vi "Event Handle Loop_Mouse Up.vi"(8 "error in (no error)":errorcluster, 10 "Coords":T1, 11 "QMenu Class in":refnum<class "QMenu Class.lvclass">) -> (0 "error out":errorcluster, 3 "QMenu Class out":refnum<class "QMenu Class.lvclass">)   [LabVIEW 2020, in "QTab.lvlib" / "QMenu Class.lvclass"]
uses:
  QMenu Class.lvclass
  <vilib>/Utility/miscctls.llb/LVPoint32TypeDef.ctl
  QMenu Class.lvclass/QMenu Class.ctl
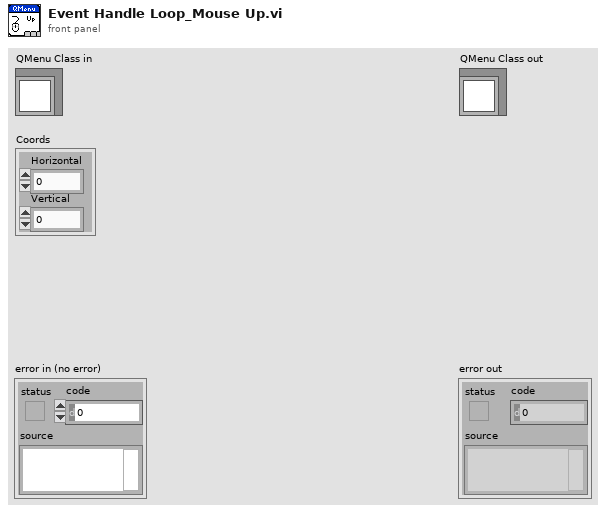
[diagram p1: front panel]
types:
  T1 = typedef "LVPoint32TypeDef.ctl" = cluster{"Horizontal":i32, "Vertical":i32}
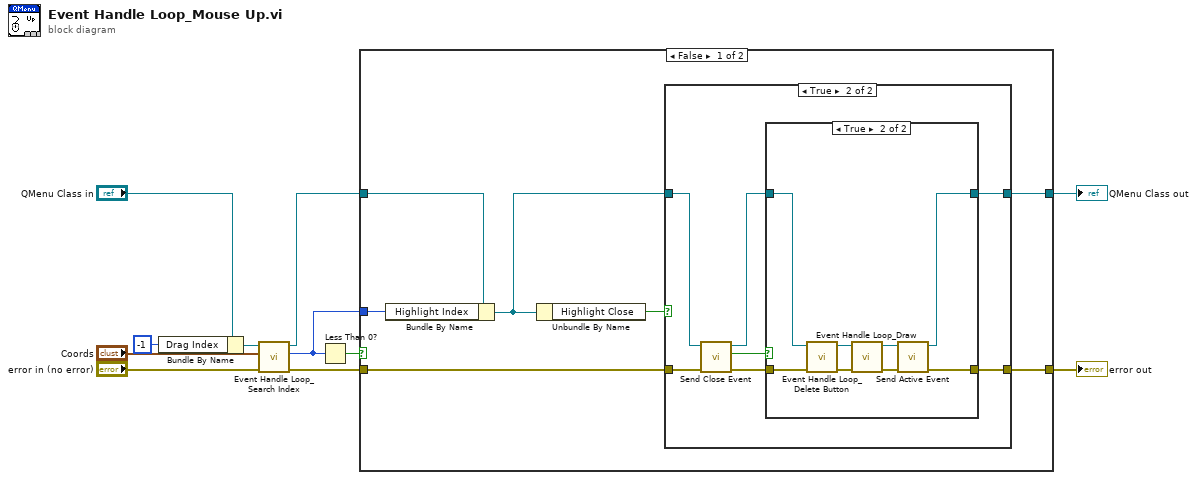
[diagram p0: block diagram]
diagram:
  n1 = Bundle By Name(cluster="QMenu Class in", "Drag Index"=-1 ("Buffer Data.Drag Index")) -> (w2:refnum<class "QMenu Class.lvclass">)
  n2 = call "Event Handle Loop_Search Index.vi"("error in (no error)"="error in (no error)", "Coords"="Coords", "QMenu Class in"=w2) -> ("error out"=w9:errorcluster, "Index"=w6:i32, "QMenu Class out"=w4:refnum<class "QMenu Class.lvclass">)  [unwired: 6 in]
  n3 = Less Than 0?(x=w6) -> (x < 0?=w8:bool)
  n4 = case shown="False" w8 {
    tunnel: w9 -> [w18 w38]
    tunnel: w4 -> [w14 w39]
    tunnel: [w17 w39] -> w7
    tunnel: w6 -> [w13 _]
    tunnel: [w15 w38] -> w5
    frame False {
      n5 = Bundle By Name(cluster=w14, "Highlight Index"=w13) -> (w16:refnum<class "QMenu Class.lvclass">)
      n6 = Unbundle By Name(w16) -> ("Highlight Close"=w12:bool)
      n7 = case shown="True" w12 {
        tunnel: w18 -> [w19 w27]
        tunnel: w16 -> [w20 w26]
        tunnel: [w20 w22] -> w17
        tunnel: [w19 w21] -> w15
        frame False {
        }
        frame True {
          n8 = call "Send Close Event.vi"("error in (no error)"=w27, "QMenu Class in"=w26) -> ("error out"=w25:errorcluster, "Confirm"=w24:bool, "QMenu Class out"=w23:refnum<class "QMenu Class.lvclass">)  [unwired: 7 in]
          n9 = case shown="True" w24 {
            tunnel: w25 -> [w29 w33]
            tunnel: w23 -> [w28 w32]
            tunnel: [w28 w35] -> w22
            tunnel: [w29 w34] -> w21
            frame False {
            }
            frame True {
              n10 = call "Event Handle Loop_Delete Button.vi"("error in (no error)"=w33, "QMenu Class in"=w32) -> ("error out"=w30:errorcluster, "QMenu Class out"=w31:refnum<class "QMenu Class.lvclass">)  [unwired: 8 in]
              n11 = call "Event Handle Loop_Draw.vi"("error in (no error)"=w30, "QMenu Class in"=w31) -> ("error out"=w37:errorcluster, "QMenu Class out"=w36:refnum<class "QMenu Class.lvclass">)  [unwired: 8 in]
              n12 = call "Send Active Event.vi"("error in (no error)"=w37, "QMenu Class in"=w36) -> ("error out"=w34:errorcluster, "QMenu Class out"=w35:refnum<class "QMenu Class.lvclass">)  [unwired: 8 in]
            }
          }
        }
      }
    }
    frame True {
    }
  }
  "error out" <- w5
  "QMenu Class out" <- w7
